vi "setTxTimestampFIFO.vi"(10 "TxTimestampFIFO":refnum<class "IReadU64FIFO.lvclass">, 11 "Modbus in":refnum<class "Modbus.lvclass">) -> (3 "Modbus out":refnum<class "Modbus.lvclass">)   [LabVIEW 2016, in "RTModbusFPGA.lvlib" / "Modbus.lvclass"]
uses:
  Modbus.lvclass
  Common_RT_FPGA/IReadU64FIFO/IReadU64FIFO.lvclass
  Modbus.lvclass/Modbus.ctl
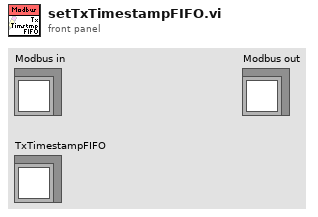
[diagram p1: front panel]
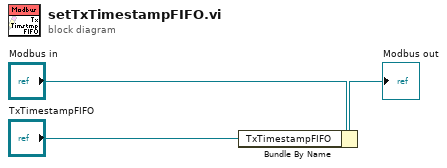
[diagram p0: block diagram]
diagram:
  n1 = Bundle By Name(cluster="Modbus in", "TxTimestampFIFO"="TxTimestampFIFO") -> (→"Modbus out":refnum<class "Modbus.lvclass">)
